vi "Update Number of Digital Channels.vi"(10 "New Number":i32, 11 "UI Data in":refnum<class "Settings UI.lvclass">) -> (3 "UI Data out":refnum<class "Settings UI.lvclass">)   [LabVIEW 2024, in "Output Sequencer.lvlib" / "Settings UI.lvclass"]
uses:
  Settings UI.lvclass
  Types/Tree Index Enum.ctl
  Settings UI.lvclass/Settings UI.ctl
  Globals/Global Tree Data.vi
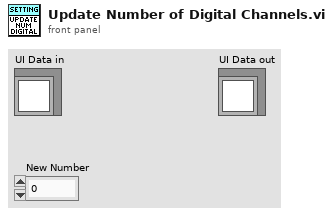
[diagram p1: front panel]
types:
  T1 = typedef "Output Sequencer.lvlib/Settings UI.lvclass/Tree Index Enum.ctl" = enum16{"General Settings", "Num Steps", "Num Analog", "Num Digital", "Show Confirmation", "Interp Priority", "Adv Timing", "Enable Conditions", "Seq Execution", "Reset Test Start", "Only When Test", "Delay After Test", "Start condition", "Re-triggering", "Stop condition", "Stop After Cycles", "Stop Values", "Default Values", "Default Analog", "Default Digital", "Steps", "Step #", "Description", "Precondition", "Duration", "Mode", "Delay Between Vals", "Analog Values", "Digital Values", "Postcondition", "On True", "On False"}
  T2 = typedef "Output Sequencer.lvlib/Settings UI.lvclass/Step Settings.ctl" = cluster{"Description":string, "Precondition":string, "Duration":dbl, "Mode":string, "Delay Between Values":dbl, "Analog Values":string[], "Digital Values":string[], "Postcondition":string, "On True":string, "On False":string}
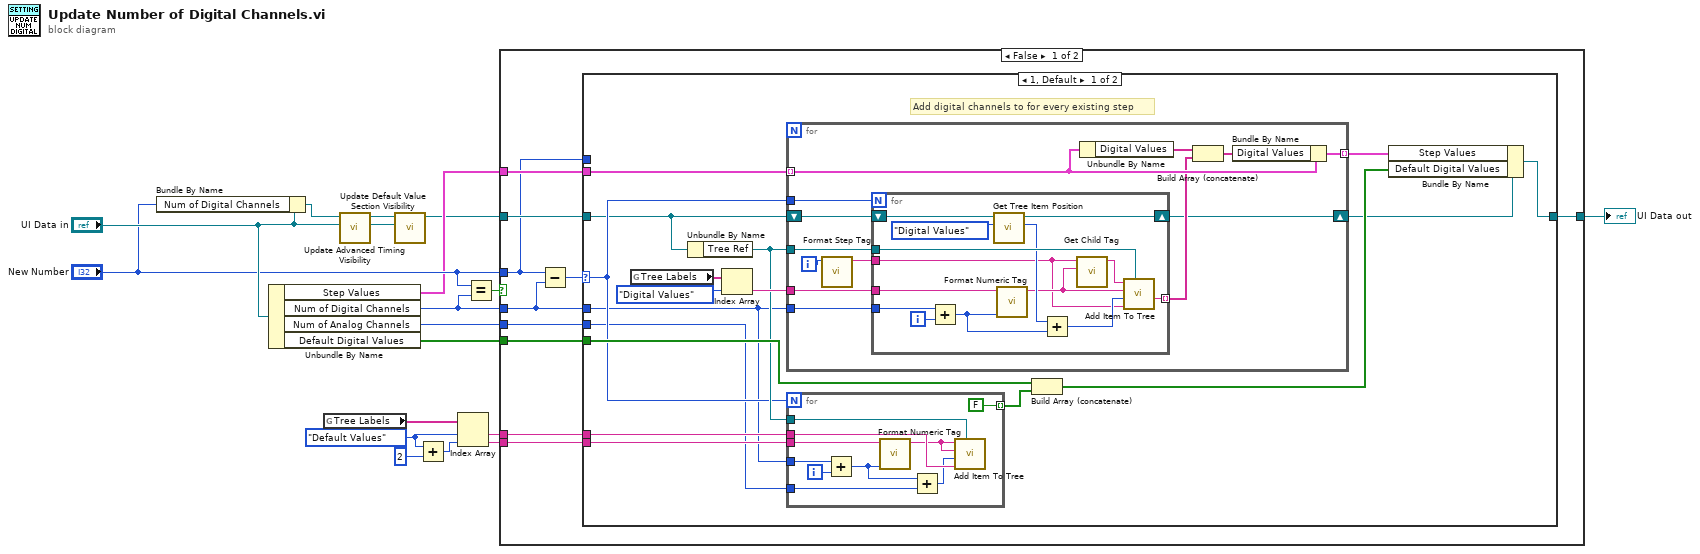
[diagram p0: block diagram]
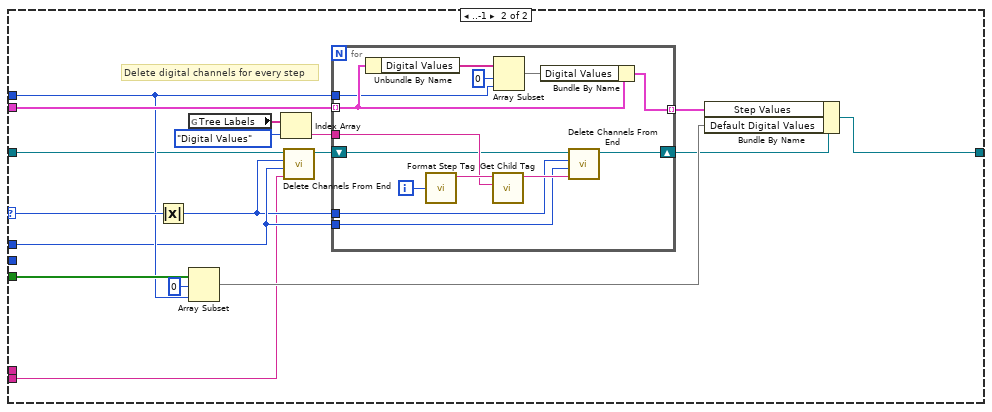
[diagram p2: hidden frame]
diagram:
  w18 = Tree_Index_Enum."Default Values" ("Tree Index Enum")
  n1 = Bundle By Name(cluster="UI Data in", "Num of Digital Channels"="New Number") -> (w2:refnum<class "Settings UI.lvclass">)
  n2 = Unbundle By Name("UI Data in") -> ("Step Values"=w5:T2[], "Num of Digital Channels"=w6:i32, "Num of Analog Channels"=w8:i32, "Default Digital Values"=w13:bool[])
  n3 = global read "Global Tree Data.vi" "Tree Labels"() -> (w9:string[])
  n4 = call "Update Advanced Timing Visibility.vi"("Previous UI Data in"="UI Data in", "New UI Data in"=w2) -> ("Previous UI Data out"=w17:refnum<class "Settings UI.lvclass">, "New UI Data out"=w15:refnum<class "Settings UI.lvclass">)  [unwired: 8 in]
  n5 = call "Update Default Value Section Visibility.vi"("Previous UI Data in"=w17, "New UI Data in"=w15) -> ("New UI Data out"=w1:refnum<class "Settings UI.lvclass">)  [unwired: 9 in]
  n6 = Add(x=w18, y=2) -> (x+y=w11:i32)
  n7 = Index Array(array=w9, index #1=w18, index #2=w11) -> (element #1=w12:string, element #2=w14:string)
  n8 = Equal?(x="New Number", y=w6) -> (x = y?=w3:bool)
  n9 = case shown="False" w3 {
    tunnel: w1 -> [w25 w114]
    tunnel: [w24 w114] -> w4
    tunnel: w6 -> [w26 _]
    tunnel: "New Number" -> [w23 _]
    tunnel: w5 -> [w27 _]
    tunnel: w8 -> [w22 _]
    tunnel: w12 -> [w21 _]
    tunnel: w14 -> [w20 _]
    tunnel: w13 -> [w19 _]
    frame False {
      n10 = Subtract(x=w23, y=w26) -> (x-y=w28:i32)
      n11 = case shown="1, Default" w28 {
        selector: w28 -> [w34 w97]
        tunnel: w27 -> [w45 w99]
        tunnel: w26 -> [w32 w89]
        tunnel: w25 -> [w31 w85]
        tunnel: [w41 w94] -> w24
        tunnel: w23 -> [_ w91]
        tunnel: w22 -> [w30 _]
        tunnel: w21 -> [w35 _]
        tunnel: w20 -> [w33 w86]
        tunnel: w19 -> [w39 w93]
        frame 1, Default {
          # "Add digital channels to for every existing step"
          n12 = global read "Global Tree Data.vi" "Tree Labels"() -> (w44:string[])
          n13 = Unbundle By Name(w31) -> ("Tree Ref"=w36:refnum<vi>)
          n14 = Index Array(array=w44, index=Tree_Index_Enum."Digital Values" ("Tree Index Enum")) -> (element=w43:string)
          n15 = for {
            tunnel: w36 -> [w68]
            tunnel: w45 -> [w64] mode=indexing
            tunnel: w32 -> [w67]
            tunnel: w34 -> [w66]
            tunnel: w43 -> [w65]
            tunnel: [w60] -> w42 mode=indexing
            shift-right: [w56] -> w29
            shift-left: w31 -> [w59]
            i -> [w58]
            n16 = call "Format Step Tag.vi"("Step Number"=w58) -> ("Tag"=w57:string)  [unwired: 10 in]
            n17 = for {
              N: w66 -> [_]
              tunnel: w68 -> [w82]
              tunnel: w67 -> [w81]
              tunnel: w65 -> [w73]
              tunnel: w57 -> [w70]
              tunnel: [w78] -> w62 mode=indexing
              shift-right: [w69] -> w56
              shift-left: w59 -> [w77]
              i -> [w80]
              n18 = Add(x=w81, y=w80) -> (x+y=w71:i32)
              n19 = call "Get Tree Item Position.vi"("Step item"=Tree_Index_Enum."Digital Values", "UI Data in"=w77) -> ("Position"=w75:i32, "UI Data out"=w69:refnum<class "Settings UI.lvclass">)  [unwired: 8 in]
              n20 = call "Format Numeric Tag.vi"("Number"=w71, "Tree label"=w73) -> ("Tag"=w72:string)  [unwired: 9 in]
              n21 = Add(x=w75, y=w71) -> (x+y=w79:i32)
              n22 = call "Get Child Tag.vi"("Child label"=w72, "Parent tag"=w70) -> ("Child tag"=w74:string)  [unwired: 9 in]
              n23 = call "Add Item To Tree.vi"("TreeControl in"=w82, "Parent Tag"=w70, "Child Position"=w79, "Left Cell String"=w72, "Child Tag in"=w74) -> ("Child Text out"=w78:string)  [unwired: 6 in]
            }
            n24 = Unbundle By Name(w64) -> ("Digital Values"=w63:string[])
            n25 = Build Array (concatenate)(w63, w62) -> (w61:string[])
            n26 = Bundle By Name(cluster=w64, "Digital Values"=w61) -> (w60:T2)
          }
          n27 = for {
            N: w34 -> [_]
            tunnel: w36 -> [w55]
            tunnel: w35 -> [w52]
            tunnel: w33 -> [w48]
            tunnel: w32 -> [w53]
            tunnel: [FALSE] -> w40 mode=indexing
            tunnel: w30 -> [w50]
            i -> [w54]
            n28 = Add(x=w53, y=w54) -> (x+y=w46:i32)
            n29 = call "Format Numeric Tag.vi"("Number"=w46, "Tree label"=w48) -> ("Tag"=w47:string)  [unwired: 9 in]
            n30 = Add(x=w46, y=w50) -> (x+y=w49:i32)
            n31 = call "Add Item To Tree.vi"("TreeControl in"=w55, "Parent Tag"=w52, "Child Position"=w49, "Left Cell String"=w47, "Child Tag in"=w47) -> ()  [unwired: 6 in, 1 out]
          }
          n32 = Build Array (concatenate)(w39, w40) -> (w38:bool[])
          n33 = Bundle By Name(cluster=w29, "Step Values"=w42, "Default Digital Values"=w38) -> (w41:refnum<class "Settings UI.lvclass">)
        }
        frame ..-1 {
          # "Delete digital channels for every step"
          n34 = Absolute Value(x=w97) -> (abs(x)=w87:i32)
          n35 = global read "Global Tree Data.vi" "Tree Labels"() -> (w98:string[])
          n36 = Array Subset(array=w93, index=0, length=w91) -> (w90:bool[])
          n37 = Index Array(array=w98, index=Tree_Index_Enum."Digital Values" ("Tree Index Enum")) -> (element=w96:string)
          n38 = call "Delete Channels From End.vi"("Channel Label"=w86, "Prior Number of Channels"=w89, "Number of Channels to Delete"=w87, "UI Data in"=w85) -> ("UI Data out"=w84:refnum<class "Settings UI.lvclass">)  [unwired: 7 in]
          n39 = for {
            tunnel: w99 -> [w113] mode=indexing
            tunnel: w89 -> [w102]
            tunnel: w87 -> [w101]
            tunnel: w96 -> [w105]
            tunnel: [w112] -> w95 mode=indexing
            tunnel: w91 -> [w109]
            shift-right: [w100] -> w83
            shift-left: w84 -> [w104]
            i -> [w107]
            n40 = Unbundle By Name(w113) -> ("Digital Values"=w111:string[])
            n41 = call "Format Step Tag.vi"("Step Number"=w107) -> ("Tag"=w106:string)  [unwired: 10 in]
            n42 = call "Get Child Tag.vi"("Child label"=w105, "Parent tag"=w106) -> ("Child tag"=w103:string)  [unwired: 9 in]
            n43 = Array Subset(array=w111, index=0, length=w109) -> (w110:string[])
            n44 = Bundle By Name(cluster=w113, "Digital Values"=w110) -> (w112:T2)
            n45 = call "Delete Channels From End.vi"("Channel Label"=w103, "Prior Number of Channels"=w102, "Number of Channels to Delete"=w101, "UI Data in"=w104) -> ("UI Data out"=w100:refnum<class "Settings UI.lvclass">)  [unwired: 7 in]
          }
          n46 = Bundle By Name(cluster=w83, "Step Values"=w95, "Default Digital Values"=w90) -> (w94:refnum<class "Settings UI.lvclass">)
        }
      }
    }
    frame True {
    }
  }
  "UI Data out" <- w4
